vi "Adb Port Reverse.vi"(8 "error in (no error)":errorcluster, 9 "remote port":u16, 10 "local port":u16, 11 "AdbBridge in":refnum<class "AdbBridge.lvclass">) -> (0 "error out":errorcluster, 3 "AdbBridge out":refnum<class "AdbBridge.lvclass">)   [LabVIEW 2016, in "AdbBridge.lvclass"]
uses:
  AdbBridge.lvclass
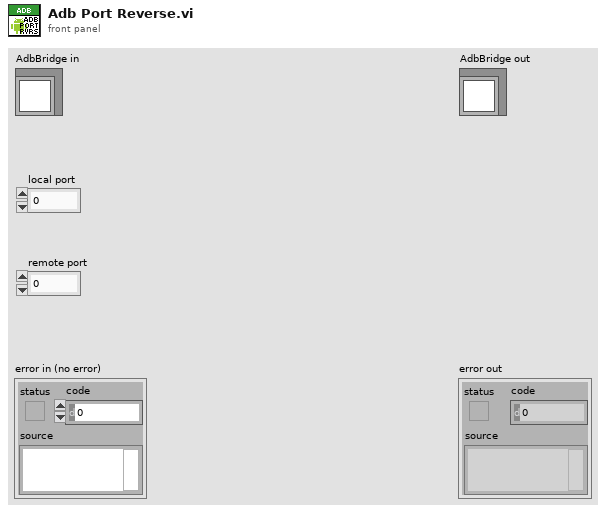
[diagram p1: front panel]
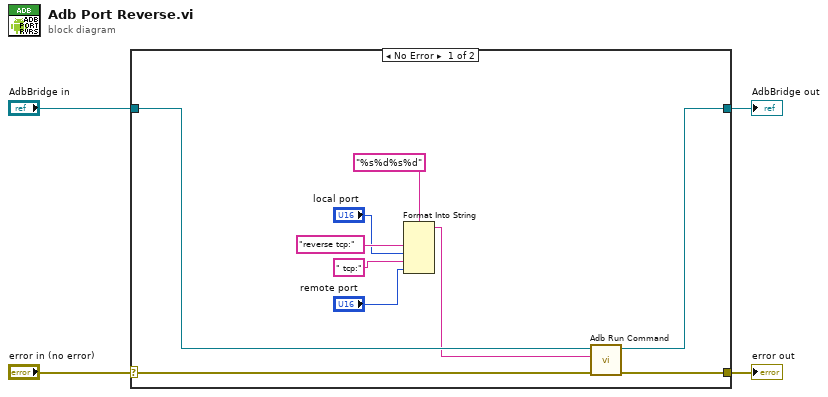
[diagram p0: block diagram]
diagram:
  n1 = case shown="No Error" "error in (no error)" {
    selector: "error in (no error)" -> [w12 w16]
    tunnel: [w11 w16] -> w3
    tunnel: [w13 w15] -> w1
    tunnel: "AdbBridge in" -> [w14 w15]
    frame No Error {
      n2 = Format Into String(format string="%s%d%s%d", "reverse tcp:" ("args"), "local port", " tcp:" ("args"), "remote port") -> (resulting string=w6:string)  [unwired: 2 in, 1 out]
      n3 = call "Adb Run Command.vi"("error in (no error)"=w12, "args"=w6, "AdbBridge in"=w14) -> ("error out"=w11:errorcluster, "AdbBridge out"=w13:refnum<class "AdbBridge.lvclass">)  [unwired: 7 in]
    }
    frame Error {
    }
  }
  "error out" <- w3
  "AdbBridge out" <- w1
